vi "FPGA_CoordCalibrationSingleApproach.vi"(4 "RetRate us":i32, 5 "AppRate us":i32, 6 "Retract":fxp<+/-,48,16>, 7 "Threshold":fxp<+/-,48,16>, 8 "Y_Dst":fxp<+/-,48,16>, 9 "Y_Start":fxp<+/-,48,16>, 10 "X_Dst":fxp<+/-,48,16>, 11 "X_Start":fxp<+/-,48,16>) -> (1 "Z_Out":fxp<+/-,48,16>, 2 "Y_Out":fxp<+/-,48,16>, 3 "X_Out":fxp<+/-,48,16>)   [LabVIEW 2024]
uses:
  <vilib>/rvi/FXPMathLib/FxpDiv/subVIs/nifxpmath_Div_SimConfig.ctl
  <vilib>/rvi/Emulation/niFpgaGetClockAttributes.vi
  <vilib>/rvi/Emulation/niFpgaSctlEmulationGetInTimedLoop.vi
  <vilib>/rvi/Emulation/niFpgaEmulationReportErrorSimple.vi
  <vilib>/rvi/Emulation/niFpgaProcessEmulError.vi
  <vilib>/rvi/Emulation/niFpgaEmulationIsFPGAContextNoSignature.vi
  <vilib>/rvi/DataTransferAndStorage/Container/Common/niFpgaContainerGetUniqueNameForEmu.vi
  <vilib>/rvi/Memory/Memory_Emulation/niFpgaMemoryEmulationCacheClearOnFirstRun.vi
  <vilib>/rvi/Memory/Memory_Emulation/nirvimemoryEmulationManagerCache_MakeExclusive.vi
  <vilib>/rvi/Memory/Memory_Emulation/niFpgaMemoryEmulationValidateCache.vi
  <vilib>/rvi/Memory/Memory_Emulation/nirvimemoryEmulationManagerCache_InsertValue.vi
  <vilib>/Utility/error.llb/Clear Errors.vi
  <vilib>/rvi/Memory/Memory_Emulation/nirvimemoryEmulationManagerCache_ReleaseExclusive.vi
  <vilib>/rvi/Memory/Memory_Emulation/nirvimemoryEmulationManagerCache_GetValue.vi
  <vilib>/rvi/Memory/Memory_Emulation/nirvimemoryEmulationManagerCache_SetValue.vi
  <vilib>/rvi/eio/common/nirviEmuTemplateMethod_errors.vi
  <vilib>/rvi/Emulation/niFpgaCriticalErrorInLSC.vi
  <vilib>/rvi/FXPMathLib/FxpDiv/simVIs/DllFxpDivTemp_sub.vi
  <vilib>/eio/utilities/niEioResolveVilibRelativePath.vi
  <vilib>/rvi/interface/RandomDataEmulation/niFpgaRandomDataHandleErrors.vi
  <vilib>/rvi/DataTransferAndStorage/Container/XNode/niFpgaContainer.xnode
  <vilib>/rvi/DataTransferAndStorage/Register/Emulation/niFpgaRegisterEmulation.vi
  <vilib>/rvi/FXPMathLib/FxpAdd/XNode/nifxpmath_Add.xnode
  <vilib>/eio/EIONode/EIONode.xnode
  <vilib>/rvi/FXPMathLib/FxpDiv/XNode/nifxpmath_Div.xnode
  <vilib>/rvi/FXPMathLib/FxpMul/XNode/nifxpmath_Multiplier.xnode
  <vilib>/rvi/FXPMathLib/FxpSub/XNode/nifxpmath_Sub.xnode
  <vilib>/rvi/interface/RandomDataEmulation/nirviRandomDataFpgaReadWriteTemplate.vi
  <vilib>/rvi/FXPMathLib/sim/FxpSim.dll
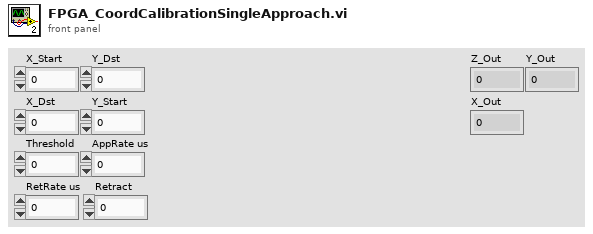
[diagram p1: front panel]
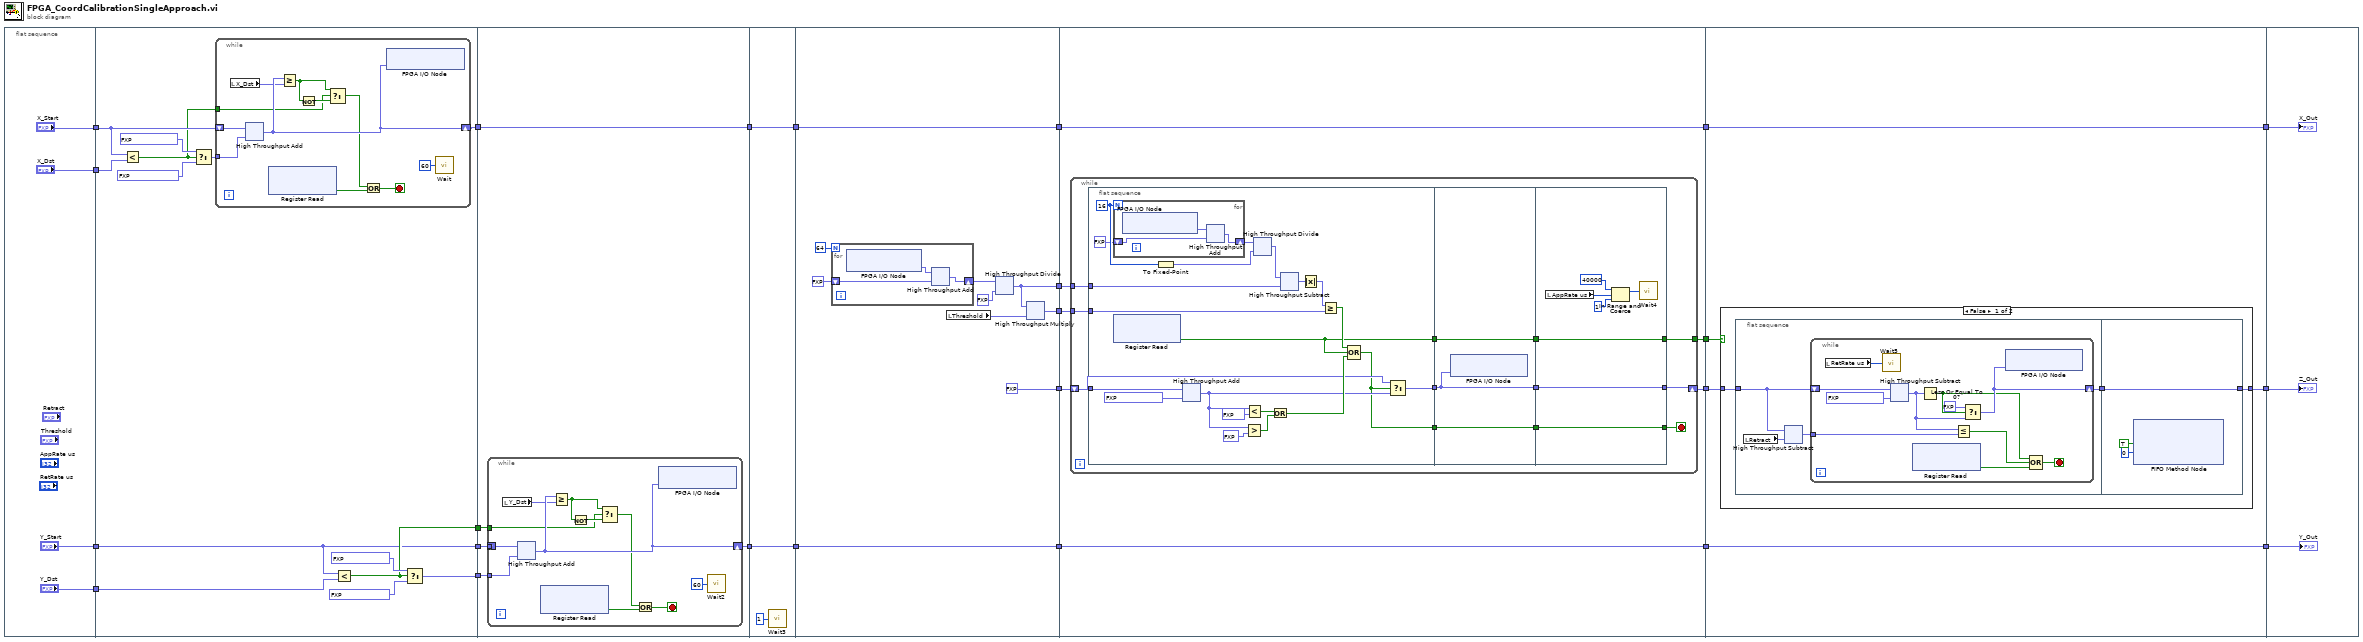
[diagram p0: block diagram]
diagram:
  n1 = flat-sequence {
    tunnel: ["X_Start"] -> w24
    tunnel: ["X_Dst"] -> w23
    tunnel: ["Y_Start"] -> w19
    tunnel: ["Y_Dst"] -> w18
    tunnel: w24 -> [w41]
    tunnel: w23 -> [w40]
    tunnel: [w33] -> w22
    tunnel: [w31] -> w21
    tunnel: [w32] -> w20
    tunnel: w19 -> [w31]
    tunnel: w18 -> [w30]
    tunnel: [w29] -> w9
    tunnel: w22 -> [w57]
    tunnel: w21 -> [w56]
    tunnel: w20 -> [w55]
    tunnel: [w54] -> w10
    tunnel: w9 -> [w54]
    tunnel: [w53] -> w5
    tunnel: [w70] -> w11
    tunnel: w10 -> [w70]
    tunnel: w5 -> [w69]
    tunnel: [w69] -> w4
    tunnel: [w76] -> w17
    tunnel: [w75] -> w16
    tunnel: [fxp<+/-,48,16> 0.0 ("Z_Start")] -> w15
    tunnel: w11 -> [w73]
    tunnel: [w73] -> w8
    tunnel: w4 -> [w72]
    tunnel: [w72] -> w3
    tunnel: w17 -> [w118]
    tunnel: w16 -> [w117]
    tunnel: w15 -> [w116]
    tunnel: [w115] -> w14
    tunnel: [w114] -> w13
    tunnel: w8 -> [w113]
    tunnel: [w113] -> w7
    tunnel: w3 -> [w112]
    tunnel: [w112] -> w2
    tunnel: w14 -> [w196]
    tunnel: w13 -> [w195]
    tunnel: [w194] -> w12
    tunnel: w7 -> [w193]
    tunnel: [w193] -> w6
    tunnel: w2 -> [w192]
    tunnel: [w192] -> w1
    tunnel: w12 -> [w221]
    tunnel: w6 -> [w220]
    tunnel: w1 -> [w219]
    frame #0 {
    }
    frame #1 {
      n2 = Less?(x=w41, y=w40) -> (x < y?=w36:bool)
      n3 = Select(t=fxp<+/-,48,16> 0.00030517578125 ("y"), s=w36, f=fxp<+/-,48,16> -0.00030517578125 ("y")) -> (s? t:f=w37:fxp<+/-,48,16>)
      n4 = while {
        shift-right: [w48] -> w29
        shift-left: w41 -> [w49]
        tunnel: w37 -> [w46]
        tunnel: w36 -> [w43]
        stop <- w50 stop-if-true
        n5 = local read "X_Dst"() -> (w47:fxp<+/-,48,16>)
        n6 = xnode ("High Throughput Add")("x"=w49, "y"=w46) -> ("x+y"=w48:fxp<+/-,48,16>)
        n7 = xnode ("Register Read")() -> ("Data"=w51:bool)  [unwired: 1 in, 1 out]
        n8 = Greater Or Equal?(x=w48, y=w47) -> (x >= y?=w44:bool)
        n9 = Not(x=w44) -> (.not. x?=w45:bool)
        n10 = Select(t=w44, s=w43, f=w45) -> (s? t:f=w42:bool)
        n11 = Or(x=w42, y=w51) -> (x .or. y?=w50:bool)
        n12 = xnode "FPGA I/O Node"("Connector0/AO0"=w48) -> ()  [unwired: 1 in, 1 out]
        n13 = call "Wait"("Count(uSec)"=u32 60) -> ()  [unwired: 1 out]
      }
      n14 = Less?(x=w31, y=w30) -> (x < y?=w33:bool)
      n15 = Select(t=fxp<+/-,48,16> 0.00030517578125 ("y"), s=w33, f=fxp<+/-,48,16> -0.00030517578125 ("y")) -> (s? t:f=w32:fxp<+/-,48,16>)
    }
    frame #2 {
      n16 = while {
        shift-right: [w64] -> w53
        shift-left: _ -> [w65]
        tunnel: w55 -> [w62]
        tunnel: w57 -> [w59]
        tunnel: w56 -> [_]
        stop <- w66 stop-if-true
        n17 = local read "Y_Dst"() -> (w63:fxp<+/-,48,16>)
        n18 = xnode ("High Throughput Add")("x"=w65, "y"=w62) -> ("x+y"=w64:fxp<+/-,48,16>)
        n19 = xnode ("Register Read")() -> ("Data"=w67:bool)  [unwired: 1 in, 1 out]
        n20 = Greater Or Equal?(x=w64, y=w63) -> (x >= y?=w60:bool)
        n21 = Not(x=w60) -> (.not. x?=w61:bool)
        n22 = Select(t=w60, s=w59, f=w61) -> (s? t:f=w58:bool)
        n23 = Or(x=w58, y=w67) -> (x .or. y?=w66:bool)
        n24 = xnode "FPGA I/O Node"("Connector0/AO1"=w64) -> ()  [unwired: 1 in, 1 out]
        n25 = call "Wait2"("Count(uSec)"=u32 60) -> ()  [unwired: 1 out]
      }
    }
    frame #3 {
      n26 = call "Wait3"("Count(mSec)"=u8 1) -> ()  [unwired: 1 out]
    }
    frame #4 {
      n27 = for {
        N: 64 -> [_]
        shift-right: [w109] -> w79
        shift-left: fxp<+/-,48,16> 0.0 -> [w110]
        n28 = xnode "FPGA I/O Node"() -> ("Connector0/AI3"=w111:fxp<+/-,27,5>)  [unwired: 1 in, 1 out]
        n29 = xnode ("High Throughput Add")("x"=w111, "y"=w110) -> ("x+y"=w109:fxp<+/-,48,16>)
      }
      n30 = local read "Threshold"() -> (w77:fxp<+/-,48,16>)
      n31 = xnode "High Throughput Divide"("x"=w79, "y"=fxp<+/-,48,16> 64.0) -> ("x/y"=w76:fxp<+/-,48,16>)
      n32 = xnode ("High Throughput Multiply")("x"=w76, "y"=w77) -> ("x*y"=w75:fxp<+/-,48,16>)
    }
    frame #5 {
      n33 = while {
        tunnel: w118 -> [w130]
        tunnel: w117 -> [w129]
        shift-right: [w119] -> w114
        shift-left: w116 -> [w126]
        tunnel: [w120] -> w115
        stop <- w121 stop-if-true
        n34 = flat-sequence {
          tunnel: w130 -> [w145]
          tunnel: w129 -> [w143]
          tunnel: [w136] -> w128
          tunnel: w126 -> [w134]
          tunnel: [w132] -> w125
          tunnel: [w131] -> w123
          tunnel: w128 -> [w184]
          tunnel: [w184] -> w127
          tunnel: w125 -> [w183]
          tunnel: [w183] -> w124
          tunnel: w123 -> [w182]
          tunnel: [w182] -> w122
          tunnel: w127 -> [w186]
          tunnel: w124 -> [w185]
          tunnel: [w187] -> w121
          tunnel: w122 -> [w187]
          tunnel: [w186] -> w120
          tunnel: [w185] -> w119
          frame #0 {
            w150 = 16
            n35 = xnode ("Register Read")() -> ("Data"=w136:bool)  [unwired: 1 in, 1 out]
            n36 = for {
              N: w150 -> [_]
              shift-right: [w179] -> w149
              shift-left: fxp<+/-,48,16> 0.0 -> [w180]
              n37 = xnode "FPGA I/O Node"() -> ("Connector0/AI3"=w181:fxp<+/-,27,5>)  [unwired: 1 in, 1 out]
              n38 = xnode ("High Throughput Add")("x"=w181, "y"=w180) -> ("x+y"=w179:fxp<+/-,48,16>)
            }
            n39 = To Fixed-Point(number=w150) -> (fixed-point=w151:fxp<+/-,48,16>)  [unwired: 1 in]
            n40 = xnode ("High Throughput Add")("x"=w134, "y"=fxp<+/-,48,16> 0.00030517578125) -> ("x+y"=w133:fxp<+/-,48,16>)
            n41 = Greater?(x=w133, y=fxp<+/-,48,16> 9.75) -> (0:w140:bool)
            n42 = Less?(x=w133, y=fxp<+/-,48,16> -0.125) -> (x < y?=w139:bool)
            n43 = xnode "High Throughput Divide"("x"=w149, "y"=w151) -> ("x/y"=w146:fxp<+/-,48,16>)
            n44 = Or(x=w139, y=w140) -> (x .or. y?=w135:bool)
            n45 = xnode "High Throughput Subtract"("x"=w146, "y"=w145) -> ("x-y"=w147:fxp<+/-,48,16>)
            n46 = Absolute Value(x=w147) -> (abs(x)=w144:fxp<+,48,16>)
            n47 = Greater Or Equal?(x=w144, y=w143) -> (x >= y?=w142:bool)
            n48 = Compound Arithmetic op=OR(w142, w136, w135) -> (w131:bool)
            n49 = Select(t=w134, s=w131, f=w133) -> (s? t:f=w132:fxp<+/-,48,16>)
          }
          frame #1 {
            n50 = xnode "FPGA I/O Node"("Connector0/AO2"=w183) -> ()  [unwired: 1 in, 1 out]
          }
          frame #2 {
            n51 = local read "AppRate us"() -> (w188:i32)
            n52 = In Range and Coerce(upper limit=40000, x=w188, lower limit=1) -> (coerced(x)=w191:i32)  [unwired: 1 out]
            n53 = call "Wait4"("Count(uSec)"=w191) -> ()  [unwired: 1 out]
          }
        }
      }
    }
    frame #6 {
      n54 = case shown="False" w196 {
        tunnel: w195 -> [w199 w218]
        tunnel: [w198 w218] -> w194
        frame False {
          n55 = flat-sequence {
            tunnel: w199 -> [w201]
            tunnel: [w200] -> w197
            tunnel: [w217] -> w198
            tunnel: w197 -> [w217]
            frame #0 {
              n56 = local read "Retract"() -> (w203:fxp<+/-,48,16>)
              n57 = xnode "High Throughput Subtract"("x"=w201, "y"=w203) -> ("x-y"=w202:fxp<+/-,48,16>)
              n58 = while {
                tunnel: w202 -> [w210]
                shift-right: [w208] -> w200
                shift-left: w201 -> [w212]
                stop <- w204 stop-if-true
                n59 = local read "RetRate us"() -> (w214:i32)
                n60 = call "Wait5"("Count(uSec)"=w214) -> ()  [unwired: 1 out]
                n61 = xnode "High Throughput Subtract"("x"=w212, "y"=fxp<+/-,48,16> 0.00030517578125) -> ("x-y"=w209:fxp<+/-,48,16>)
                n62 = xnode ("Register Read")() -> ("Data"=w207:bool)  [unwired: 1 in, 1 out]
                n63 = Less Or Equal To 0?(x=w209) -> (x <= 0?=w205:bool)
                n64 = Less Or Equal?(x=w209, y=w210) -> (x <= y?=w206:bool)
                n65 = Select(t=fxp<+/-,48,16> 0.0, s=w205, f=w209) -> (s? t:f=w208:fxp<+/-,48,16>)
                n66 = xnode "FPGA I/O Node"("Connector0/AO2"=w208) -> ()  [unwired: 1 in, 1 out]
                n67 = Compound Arithmetic op=OR(w205, w206, w207) -> (w204:bool)
              }
            }
            frame #1 {
              n68 = xnode ("FIFO Method Node")("Element"=TRUE, "Timeout"=0) -> ()  [unwired: 1 in, 2 out]
            }
          }
        }
        frame True {
        }
      }
    }
    frame #7 {
      "Z_Out" <- w221
      "X_Out" <- w220
      "Y_Out" <- w219
    }
  }
